vi "Finish Read.vi"(8 "error in (no error)":errorcluster, 11 "WebSocket Client in":refnum<class "WebSocket Client.lvclass">) -> (0 "error out":errorcluster, 1 "Format":T1, 2 "Payload":string, 3 "WebSocket Client out":refnum<class "WebSocket Client.lvclass">)   [LabVIEW 2020, in "HTTP Server.lvlib" / "WebSocket Client.lvclass"]
uses:
  WebSocket Client.lvclass
  WebSocket Client.lvclass/WebSocket Client.ctl
  OpCode.ctl
  Message Frame.ctl
  WebSocket Format.ctl
  HTTP Server.lvlib
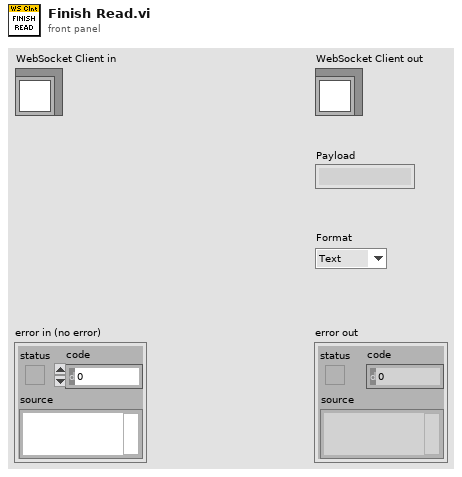
[diagram p1: front panel]
types:
  T1 = typedef "HTTP Server.lvlib/WebSocket Format.ctl" = enum16{"Text", "Binary"}
  T2 = typedef "HTTP Server.lvlib/WebSocket Client.lvclass/Message Frame.ctl" = cluster{"FIN":bool, "RSV1":bool, "RSV2":bool, "RSV3":bool, "MASK":bool, "OpCode":T3, "Length":u64, "MaskingKey":u8[], "Payload":string}
  T3 = typedef "HTTP Server.lvlib/WebSocket Client.lvclass/OpCode.ctl" = enum8{"Continuation", "Text", "Binary", "Reserved3", "Reserved4", "Reserved5", "Reserved6", "Reserved7", "Close", "Ping", "Pong", "ReservedB", "ReservedC", "ReservedD", "ReservedE", "ReservedF"}
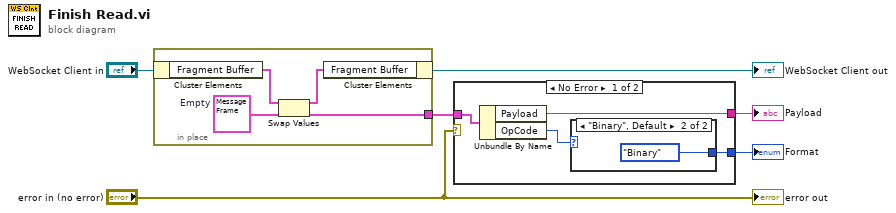
[diagram p0: block diagram]
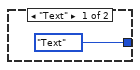
[diagram p2: hidden frame]
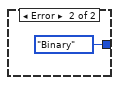
[diagram p3: hidden frame]
diagram:
  n1 = in-place {
    in-place-border: [w7] -> w6
    w9 = T2 {"FIN"=FALSE, "RSV1"=FALSE, "RSV2"=FALSE, "RSV3"=FALSE, "MASK"=FALSE, "OpCode"=enum."Continuation", "Length"=0, "MaskingKey"=[], "Payload"=""}  # Empty
    n2 = in-place-cluster #1("WebSocket Client in") -> ("Fragment Buffer"=w10:T2)
    n3 = Swap Values(12:w10, 14:w9) -> (1:w8:T2, 3:w7:T2)  [unwired: 1 in]
    n4 = in-place-cluster #1("Fragment Buffer"=w8) -> (→"WebSocket Client out":refnum<class "WebSocket Client.lvclass">)
  }
  n5 = case shown="No Error" "error in (no error)" {
    tunnel: w6 -> [w14 _]
    tunnel: [w13 _] -> w2
    tunnel: [w11 WebSocket_Format."Binary" ("Format")] -> w1
    frame No Error {
      n6 = Unbundle By Name(w14) -> ("Payload"=w13:string, "OpCode"=w12:T3)
      n7 = case shown="\"Binary\", Default" w12 {
        tunnel: [WebSocket_Format."Text" ("Format") WebSocket_Format."Binary" ("Format")] -> w11
        frame "Text" {
        }
        frame "Binary", Default {
        }
      }
    }
    frame Error {
    }
  }
  "Payload" <- w2
  "Format" <- w1
  "error out" <- "error in (no error)"
